vi "EventosWebServer.vi"(8 "error in (no error)":errorcluster, 10 "Datos":T1={"Imei"="359772033694416", "Evento"="Automático", "Lat"="-2.884192", "Lon"="-79.012285", "F_H_eve"=timestamp(3439900564 s since 1904-01-01), "F_H_rec"=timestamp(3447157248.23 s since 1904-01-01)}, 11 "Refnum in":T2) -> (0 "error out":errorcluster, 3 "Refnum out":T2)   [LabVIEW 2012]
uses:
  <vilib>/addons/database/Connection.llb/Conn ObjectReference.ctl
  <vilib>/addons/database/Auxilliary.llb/DB Tools Parameter Info.ctl
  <vilib>/addons/database/Auxilliary.llb/DB Tools DataTypes.ctl
  <vilib>/addons/database/Auxilliary.llb/DB Tools Parameter Dir.ctl
  <vilib>/addons/database/Connection.llb/Conn Execute.vi
  <vilib>/addons/database/Recordset.llb/Rec Get Recordset Properties (R).vi
  <vilib>/addons/database/Recordset.llb/Rec Fetch String Data (R).vi
  <vilib>/addons/database/Recordset.llb/Rec Fetch Integer Data (R).vi
  <vilib>/addons/database/Recordset.llb/Rec Destroy - Connection.vi
  <vilib>/addons/database/Auxilliary.llb/DB Tools Format Datetime String (Time Stamp).vi
  <vilib>/addons/database/Command.llb/Cmd Set Parameter Value (C).vi
  <vilib>/addons/database/Command.llb/Cmd Execute.vi
  <vilib>/addons/database/Recordset.llb/Rec Destroy - Command.vi
  <vilib>/addons/database/Command.llb/Cmd Delete.vi
  <vilib>/addons/database/NI_Database_API.lvlib
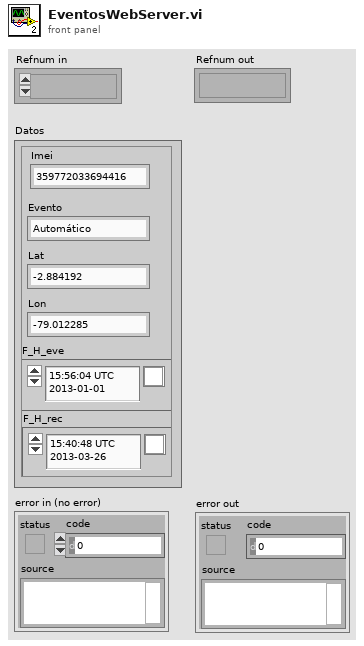
[diagram p1: front panel]
types:
  T1 = cluster{"Imei":string, "Evento":string, "Lat":string, "Lon":string, "F_H_eve":timestamp, "F_H_rec":timestamp}
  T2 = typedef "NI_Database_API.lvlib/Conn ObjectReference.ctl" = refnum<k1>
  T3 = enum16{"POC", "Imei", "Evento", "Lat", "Lon", "F_H_eve", "F_H_rec", "AVL_N", "AVL_pass", "Propietario", "Razon_Social", "Direccion", "Propietario_N", "Ciudad", "Marca", "Ruta", "N_Ruta", "Auditor", "Auditor_ST", "Auditor_N"}
  T4 = enum16{"POC", "Imei", "Evento", "Lat", "Lon", "F_H_eve", "F_H_rec", "AVL_N", "AVL_pass", "Propietario", "Razon_Social", "Direccion", "Propietario_N", "Ciudad", "Marca", "Ruta", "N_Ruta", "Auditor", "Auditor_N"}
  T5 = typedef "NI_Database_API.lvlib/DB Tools Parameter Info.ctl" = cluster{"parameter name":string, "type":T6, "direction":T7, "value":variant}
  T6 = typedef "NI_Database_API.lvlib/DB Tools DataTypes.ctl" = enum16{"String", "Long (I32)", "Single (SGL)", "Double (DBL)", "Date/Time", "Binary"}
  T7 = typedef "NI_Database_API.lvlib/DB Tools Parameter Dir.ctl" = enum32{"Input", "Output", "Input/Output", "Return Value"}
  T8 = typedef "NI_Database_API.lvlib/Rec ObjectReference.ctl" = refnum<k1>
  T9 = typedef "NI_Database_API.lvlib/Cmd ObjectReference.ctl" = refnum<k1>
  T10 = typedef "NI_Database_API.lvlib/Cmd-Rec Object Reference.ctl" = refnum<k1>
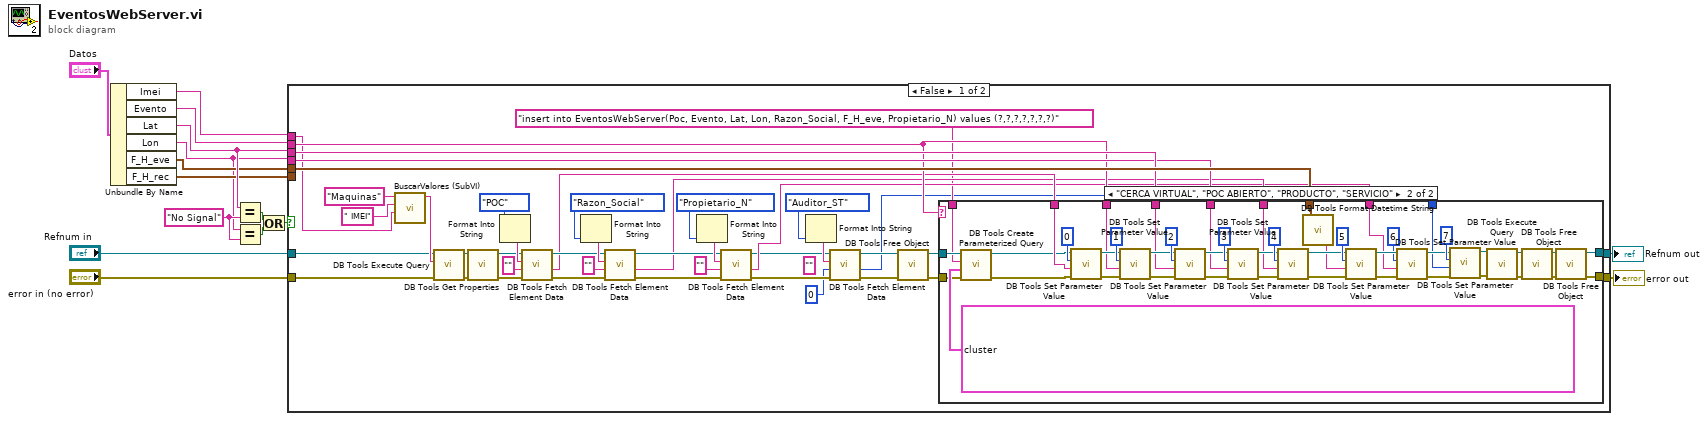
[diagram p0: block diagram]
diagram:
  w12 = "No Signal" ("y")
  n1 = Unbundle By Name("Datos") -> ("Imei"=w11:string, "Evento"=w3:string, "Lat"=w10:string, "Lon"=w7:string, "F_H_eve"=w9:timestamp, "F_H_rec"=w8:timestamp)
  n2 = Equal?(x=w10, y=w12) -> (x = y?=w14:bool)
  n3 = Equal?(x=w7, y=w12) -> (x = y?=w15:bool)
  n4 = Or(x=w14, y=w15) -> (x .or. y?=w13:bool)
  n5 = case shown="False" w13 {
    tunnel: [w58 w107] -> w2
    tunnel: [w57 w106] -> w1
    tunnel: w8 -> [_ _]
    tunnel: w9 -> [w56 _]
    tunnel: w7 -> [w54 _]
    tunnel: w10 -> [w55 _]
    tunnel: w3 -> [w53 _]
    tunnel: w11 -> [w28 _]
    tunnel: "Refnum in" -> [w32 w107]
    tunnel: "error in (no error)" -> [w31 w106]
    frame False {
      (unwired) "" ("type")
      n6 = call "BuscarValores (SubVI).vi"("="=w28, "Columna"=" IMEI" ("Substring"), "Tabla"="Maquinas" ("table")) -> ("String"=w47:string)  [unwired: 8 in]
      n7 = call-poly <vilib>:"DB Tools Execute Query.vi"("error in (no error)"=w31, "SQL query"=w47, "connection reference"=w32) -> ("error out"=w50:errorcluster, "recordset reference"=w51:T8)  [unwired: 5 in]
      n8 = call-poly <vilib>:"DB Tools Get Properties.vi"("error in (no error)"=w50, "recordset reference"=w51) -> ("error out"=w37:errorcluster, "recordset reference out"=w38:T8)  [unwired: 3 in, 1 out]
      n9 = Format Into String(T4."POC") -> (resulting string=w46:string)  [unwired: 3 in, 1 out]
      n10 = call-poly <vilib>:"DB Tools Fetch Element Data.vi"("error in (no error)"=w37, "type"="", "column index"=w46, "recordset reference"=w38) -> ("error out"=w40:errorcluster, "data"=w27:string, "recordset reference out"=w41:T8)  [unwired: 3 in]
      n11 = Format Into String(T4."Razon_Social") -> (resulting string=w42:string)  [unwired: 3 in, 1 out]
      n12 = call-poly <vilib>:"DB Tools Fetch Element Data.vi"("error in (no error)"=w40, "type"="", "column index"=w42, "recordset reference"=w41) -> ("error out"=w33:errorcluster, "data"=w26:string, "recordset reference out"=w34:T8)  [unwired: 3 in]
      n13 = Format Into String(T4."Propietario_N") -> (resulting string=w36:string)  [unwired: 3 in, 1 out]
      n14 = call-poly <vilib>:"DB Tools Fetch Element Data.vi"("error in (no error)"=w33, "type"="", "column index"=w36, "recordset reference"=w34) -> ("error out"=w19:errorcluster, "data"=w25:string, "recordset reference out"=w18:T8)  [unwired: 3 in]
      n15 = Format Into String(T3."Auditor_ST") -> (resulting string=w23:string)  [unwired: 3 in, 1 out]
      n16 = call-poly <vilib>:"DB Tools Fetch Element Data.vi"("error in (no error)"=w19, "type"=0, "column index"=w23, "recordset reference"=w18) -> ("error out"=w20:errorcluster, "data"=w17:i32, "recordset reference out"=w21:T8)  [unwired: 3 in]
      n17 = call-poly <vilib>:"DB Tools Free Object.vi"("error in (no error)"=w20, "recordset reference"=w21) -> ("error out"=w29:errorcluster, "connection reference"=w30:T2)  [unwired: 8 in]
      n18 = case shown="\"CERCA VIRTUAL\", \"POC ABIERTO\", \"PRODUCTO\", \"SERVICIO\"" w53 {
        tunnel: w29 -> [w59 w88]
        tunnel: w30 -> [w60 w87]
        tunnel: [w60 w86] -> w58
        tunnel: [w59 w85] -> w57
        tunnel: w56 -> [_ w76]
        tunnel: w53 -> [_ w75]
        tunnel: w55 -> [_ w74]
        tunnel: w54 -> [_ w73]
        tunnel: w27 -> [_ w72]
        tunnel: w26 -> [_ w71]
        tunnel: w25 -> [_ w70]
        tunnel: "insert into EventosWebServer(Poc, Evento, Lat, Lon, Razon_Social, F_H_eve, Propietario_N) values (?,?,?,?,?,?,?)" ("SQL query") -> [_ w69]
        tunnel: w17 -> [_ w63]
        frame "", Default {
        }
        frame "CERCA VIRTUAL", "POC ABIERTO", "PRODUCTO", "SERVICIO" {
          n19 = call <vilib>:"DB Tools Create Parameterized Query.vi"("error in (no error)"=w88, "parameters"=T5[] [{"parameter name"="Poc", "type"=enum."String", "direction"=enum."Input", "value"=variant}, {"parameter name"="Evento", "type"=enum."String", "direction"=enum."Input", "value"=variant}, {"parameter name"="Lat", "type"=enum."String", "direction"=enum."Input", "value"=variant}, {"parameter name"="Lon", "type"=enum."String", "direction"=enum."Input", "value"=variant}, {"parameter name"="Razon_Social", "type"=enum."String", "direction"=enum."Input", "value"=variant}, {"parameter name"="F_H_eve", "type"=enum."Date/Time", "direction"=enum."Input", "value"=variant}, {"parameter name"="Propietario_N", "type"=enum."String", "direction"=enum."Input", "value"=variant}, {"parameter name"="Auditor_ST", "type"=enum."Single (SGL)", "direction"=enum."Input", "value"=variant}], "SQL query"=w69, "connection reference"=w87) -> ("error out"=w61:errorcluster, "command reference"=w62:T9)  [unwired: 3 in, 1 out]
          n20 = call-poly <vilib>:"DB Tools Set Parameter Value.vi"("error in (no error)"=w61, "value"=w72, "parameter index"=0, "command reference"=w62) -> ("error out"=w90:errorcluster, "command reference out"=w91:T9)  [unwired: 4 in]
          n21 = call-poly <vilib>:"DB Tools Set Parameter Value.vi"("error in (no error)"=w90, "value"=w75, "parameter index"=1, "command reference"=w91) -> ("error out"=w97:errorcluster, "command reference out"=w98:T9)  [unwired: 4 in]
          n22 = call-poly <vilib>:"DB Tools Set Parameter Value.vi"("error in (no error)"=w97, "value"=w74, "parameter index"=2, "command reference"=w98) -> ("error out"=w96:errorcluster, "command reference out"=w95:T9)  [unwired: 4 in]
          n23 = call-poly <vilib>:"DB Tools Set Parameter Value.vi"("error in (no error)"=w96, "value"=w73, "parameter index"=3, "command reference"=w95) -> ("error out"=w100:errorcluster, "command reference out"=w99:T9)  [unwired: 4 in]
          n24 = call-poly <vilib>:"DB Tools Set Parameter Value.vi"("error in (no error)"=w100, "value"=w71, "parameter index"=4, "command reference"=w99) -> ("error out"=w79:errorcluster, "command reference out"=w80:T9)  [unwired: 4 in]
          n25 = call-poly <vilib>:"DB Tools Format Datetime String.vi"("time stamp"=w76) -> ("date/time string"=w78:string)
          n26 = call-poly <vilib>:"DB Tools Set Parameter Value.vi"("error in (no error)"=w79, "value"=w78, "parameter index"=5, "command reference"=w80) -> ("error out"=w84:errorcluster, "command reference out"=w83:T9)  [unwired: 4 in]
          n27 = call-poly <vilib>:"DB Tools Set Parameter Value.vi"("error in (no error)"=w84, "value"=w70, "parameter index"=6, "command reference"=w83) -> ("error out"=w66:errorcluster, "command reference out"=w67:T9)  [unwired: 4 in]
          n28 = call-poly <vilib>:"DB Tools Set Parameter Value.vi"("error in (no error)"=w66, "value"=w63, "parameter index"=7, "command reference"=w67) -> ("error out"=w64:errorcluster, "command reference out"=w65:T9)  [unwired: 4 in]
          n29 = call-poly <vilib>:"DB Tools Execute Query.vi"("error in (no error)"=w64, "command reference"=w65) -> ("error out"=w92:errorcluster, "command-recordset reference"=w93:T10)  [unwired: 6 in]
          n30 = call-poly <vilib>:"DB Tools Free Object.vi"("error in (no error)"=w92, "command-recordset reference"=w93) -> ("error out"=w94:errorcluster, "command reference"=w77:T9)  [unwired: 8 in]
          n31 = call-poly <vilib>:"DB Tools Free Object.vi"("error in (no error)"=w94, "command reference"=w77) -> ("error out"=w85:errorcluster, "connection reference"=w86:T2)  [unwired: 8 in]
        }
      }
    }
    frame True {
    }
  }
  "error out" <- w1
  "Refnum out" <- w2
